vi "AlliGator Close White Light Image.vi"(7 "AlliGator Ctrl Refnums":T1, 8 "error in (no error)":errorcluster, 11 "AlliGator IV DVR in":refnum<data-value>) -> (0 "error out":errorcluster, 1 "Message":string, 3 "AlliGator IV DVR out":refnum<data-value>)   [LabVIEW 2021, in "AlliGator Files.lvlib"]
doc: "Clears White Light Image structure."
uses:
  AlliGator Files.lvlib
  Internal Variables/AlliGator Internal Variables v2.ctl
  <vilib>/vision/Image Controls.llb/IMAQ Image.ctl
  Internal Variables/AlliGator Gate Image Set.ctl
  AlliGator FLI Dataset Type.ctl
  AlliGator Data Series Type.ctl
  Dual-Channel Datasets/AlliGator Dataset Channel.ctl
  Settings/AlliGator Gate Arithmetic.ctl
  Source Image/AlliGator Displayed Image.ctl
  Image/Named ROI Description.ctl
  Phasor Graph/AlliGator Decay Metadata v3.ctl
  Decay Analysis/Decay Preprocessing/AlliGator Decay Background Subtraction Info.ctl
  Decay Analysis/Decay Preprocessing/AlliGator Baseline Subtraction Method.ctl
  Graphs/XY Graph/XY Graph Plot Shift Parameters.ctl
  Graphs/XY Graph/XY Graph Plot Shift Method.ctl
  Decay Analysis/Decay Preprocessing/AlliGator Decay Extrapolation Parameters.ctl
  Phasor/Calibration Phasor (m, phi).ctl
  Phasor/Phasor Reference Series.ctl
  Phasor/Phasor Calibration Map v2.ctl
  Phasor/Phasor (g, s).ctl
  Phasor Graph/AlliGator Raw Phasor Plot Data v5.ctl
  Phasor/Phasor Standard Deviation Options.ctl
  Phasor Plot/AlliGator Phasor Multi-Harmonic Data.ctl
  Phasor/Phasor Harmonic Data.ctl
  Decay Fit Parameter Map/AlliGator Decay Fit Options & Parameters v3.ctl
  Fits/IRF(X)PSED/Decay Fit Options v3.ctl
  Fits/Decay Convolution/Decay Model.ctl
  Fits/Residual Type.ctl
  Fits/IRF(X)PSED/Fit Weights Type.ctl
  Fits/Non-linear Fitting Method v2.ctl
  Fits/Fit Calculation Method.ctl
  Fits/Non-linear Fitting Algorithm.ctl
  Decay Analysis/Decay Fit/AlliGator Decay Fit Parameter Constraints 2.ctl
  Fits/IRF(X)PSED/Decay Fit Parameters In List.ctl
  Fits/IRF(X)PSED/MLE Baseline Offset Type.ctl
  Decay Analysis/Decay Preprocessing/AlliGator Decay Preprocessing Parameters.ctl
  Fits/IRF(X)PSED/Decay Fit Parameters & Derived Quantities List v2.ctl
  Fits/IRF(X)PSED/Decay Fit Result Constraint.ctl
  Decay Fit Parameter Map/AlliGator Parameter Maps Data.ctl
  GUI/AlliGator Ctrl Refnums.ctl
  GUI/AlliGator Other Ctrl Refnums.ctl
  GUI/AlliGator State Indicator.ctl
  GUI/AlliGator Main Window Tabs.ctl
  GUI/AlliGator Phasor Plot Ctrl Refnums.ctl
  GUI/AlliGator Phasor Graph Ctrl Refnums.ctl
  Phasor/Phasor Calibration Type.ctl
  GUI/AlliGator Dataset Ctrl Refnums.ctl
  GUI/AlliGator Registered Events Ctrl Refnums.ctl
  GUI/AlliGator Image Histogram Control Refnums.ctl
  Histograms/Linear Histogram Options.ctl
  Histograms/Histogram Bin Option.ctl
  Histograms/Histogram Bin Position.ctl
  Decay Fit Parameter Map/AlliGator Decay Fit Map Control Refnums.ctl
  Parameter Map/AlliGator Parameter Map Control Refnums.ctl
  Phasor/Phasor.lvlib
  Image/Image.lvlib
  Decay Analysis/Decay Preprocessing/AlliGator Decay Preprocessing.lvlib
  Phasor Graph/AlliGator Phasor Graph.lvlib
  Internal Variables/AlliGator Internal Variables.lvlib
  Phasor Plot/AlliGator Phasor Plot.lvlib
  Source Image/AlliGator Source Image.lvlib
  Fits/Fits.lvlib
  Decay Analysis/Decay Fit/AlliGator Decay Fit.lvlib
  Decay Fit Parameter Map/AlliGator Decay Fit Parameter Map.lvlib
  Settings/AlliGator Settings.lvlib
  Dual-Channel Datasets/AlliGator Dual-Channel Datasets.lvlib
  GUI/AlliGator GUI.lvlib
  Histograms/Histogram Window.lvlib
  Graphs/XY Graph/XY Graph Add-Ons.lvlib
  Parameter Map/AlliGator Parameter Map.lvlib
panel:
  # "see the AlliGator License on the block diagram (Ctrl+E or Window:Show Block Diagram)"
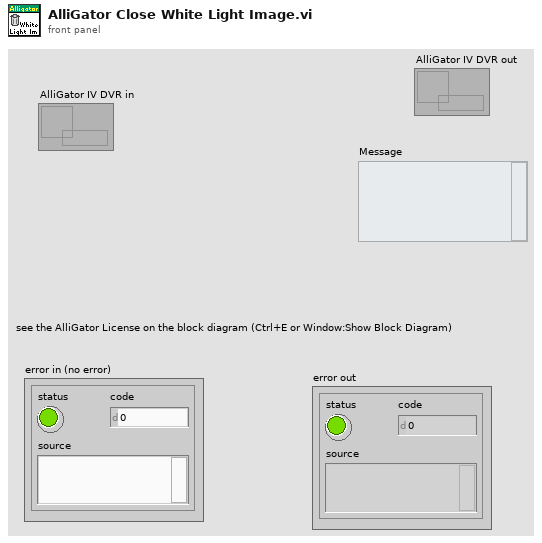
[diagram p1: front panel]
types:
  T1 = typedef "AlliGator GUI.lvlib/AlliGator Ctrl Refnums.ctl" = cluster{"Other AlliGator Ctrl Refnums":T2, "Phasor Plot Ctrl Refnums":T3, "Phasor Graph Ctrl Refnums":T4, "Dataset Control Refnums":T5, "Registered Events Ctrl Refnums":T6, "Image Histogram Ctrl Refnums":T7, "Decay Fit Map Ctrl Refnums":T8, "Parameter Map Ctrl Refnums":T9}
  T2 = typedef "AlliGator GUI.lvlib/AlliGator Other Ctrl Refnums.ctl" = cluster{"State Indicators":refnum<vi>, " Progress Bar":refnum<vi>, "Decay Graph Active":refnum<vi>, "Decay Statistics Bin":refnum<vi>, "Time Step":refnum<vi>, "Use File Timestamp":refnum<vi>, "Tab Control":refnum<vi>, "CPU":refnum<vi>, "Abort Fit":refnum<vi>, "Dataset File/Folder Path":refnum<vi>, "Abort ROI Creation":refnum<vi>, "Event LED":refnum<vi>, "Dataset File/Folder Path 2":refnum<vi>, "Dataset File/Folder Path 3":refnum<vi>, "Dataset File/Folder Path 4":refnum<vi>, "Dataset File/Folder Path 5":refnum<vi>, "Dataset File/Folder Path 6":refnum<vi>, "Dataset File/Folder Path 7":refnum<vi>, "Dataset File/Folder Path 8":refnum<vi>, "Dataset File/Folder Path 9":refnum<vi>, "Dataset File/Folder Path 10":refnum<vi>, "Dataset File/Folder Path 11":refnum<vi>}
  T3 = typedef "AlliGator GUI.lvlib/AlliGator Phasor Plot Ctrl Refnums.ctl" = cluster{"Phasor Ratio":refnum<vi>, "Modulus Lifetime":refnum<vi>, "Phasor at cursor (m, phi)":refnum<vi>, "Phase Lifetime":refnum<vi>, "Phasor at cursor (g, s)":refnum<vi>, "Phasor Plor Average Lifetime":refnum<vi>, "Phasor Plot Active":refnum<vi>, "Save Phasor Plot":refnum<vi>, "Image Overlay Color":refnum<vi>, "Phasor Plot Color Scale":refnum<vi>, "Reference 1 Button":refnum<vi>, "Reference 2 Button":refnum<vi>, "True Phasor Plot Value":refnum<vi>}
  T4 = typedef "AlliGator GUI.lvlib/AlliGator Phasor Graph Ctrl Refnums.ctl" = cluster{"Phasor Ratio":refnum<vi>, "Modulus Lifetime":refnum<vi>, "Phasor at cursor (m, phi)":refnum<vi>, "Phase Lifetime":refnum<vi>, "Phasor at cursor (g, s)":refnum<vi>, "Phasor Graph Average Lifetime":refnum<vi>, "Phasor Graph Active":refnum<vi>, "Save Phasor Graph":refnum<vi>, "Phasor Frame Slide":refnum<vi>, "Single Step Phasor":refnum<vi>, "Calibration Type":refnum<vi>, "Show Line":refnum<vi>, "Phase Lifetime 1":refnum<vi>, "Phase Lifetime 2":refnum<vi>, "Phasor Graph Frequency":refnum<vi>, "Phasor Reference 1 Control":refnum<vi>, "Phasor Reference 2 Control":refnum<vi>, "Calibration Lifetime":refnum<vi>, "Phase Lifetime SDV":refnum<vi>, "Average Lifetime SDV":refnum<vi>, "Phasor Ratio SDV":refnum<vi>, "Modulus Lifetime SDV":refnum<vi>}
  T5 = typedef "AlliGator GUI.lvlib/AlliGator Dataset Ctrl Refnums.ctl" = cluster{"Current Data":refnum<vi>, "Gate Image Slide":refnum<vi>, "Time Point Slide":refnum<vi>, "Current Time Stamp":refnum<vi>, "Save Image":refnum<vi>, "Displayed Image":refnum<vi>, "Overlay Mode":refnum<vi>, "Phasor Overlay Color":refnum<vi>, "Image Color Scale":refnum<vi>, "Use ROI as Search Area":refnum<vi>, "Source Image ROI Color":refnum<vi>, "True Pixel Value":refnum<vi>}
  T6 = typedef "AlliGator GUI.lvlib/AlliGator Registered Events Ctrl Refnums.ctl" = cluster{"Time Point Slider":refnum<vi>, "Phasor Plot Display Range":refnum<vi>, "Decay Graph":refnum<vi>, "Decay Statistics Graph":refnum<vi>, "Intensity Time Trace":refnum<vi>, "Phasor Graph":refnum<vi>, "Phasor Ratio Graph":refnum<vi>, "Lifetime Graph":refnum<vi>, "Phasor Plot Display":refnum<vi>, "Source Image Display":refnum<vi>, "Decay Fit Parameter Map Display Range":refnum<vi>, "Decay Fit Parameter Map Display":refnum<vi>, "Parameter Map Display Range":refnum<vi>, "Parameter Map Display":refnum<vi>, "Phasor Plot Display Range":refnum<vi>}
  T7 = typedef "AlliGator GUI.lvlib/AlliGator Image Histogram Control Refnums.ctl" = cluster{"Image Histogram":refnum<vi>, "Image Histogram Options":refnum<vi>, "Image Histogram Active":refnum<vi>, "Image Histogram Upper Percentile":refnum<vi>, "Image Histogram Lower Percentile":refnum<vi>, "Auto-Adjust Contrast":refnum<vi>}
  T8 = typedef "AlliGator Decay Fit Parameter Map.lvlib/AlliGator Decay Fit Map Control Refnums.ctl" = cluster{"Decay Fit Parameter Map Color Scale":refnum<vi>, "Decay Fit Parameter":refnum<vi>, "Max Parameter":refnum<vi>, "Min Parameter":refnum<vi>, "Decay Fit Parameter Map Display":refnum<vi>, "Decay Fit Parameter Map Display Range":refnum<vi>, "Decay Parameter Map X":refnum<vi>, "Decay Parameter Map Y":refnum<vi>, "Decay Parameter Map Value":refnum<vi>}
  T9 = typedef "AlliGator Parameter Map.lvlib/AlliGator Parameter Map Control Refnums.ctl" = cluster{"Parameter Map Color Scale":refnum<vi>, "Map Parameter":refnum<vi>, "Max Parameter":refnum<vi>, "Min Parameter":refnum<vi>, "Parameter Map Display":refnum<vi>, "Parameter Map Display Range":refnum<vi>, "Parameter Map Set":refnum<vi>, "Parameter Map X":refnum<vi>, "Parameter Map Y":refnum<vi>, "Parameter Map Value":refnum<vi>}
  T10 = typedef "IMAQ Image.ctl" = refnum<image>
  T11 = typedef "AlliGator Internal Variables.lvlib/AlliGator Internal Variables v2.ctl" = cluster{"----------------------------- Images -----------------------------":u8, "Displayed Image":T10, "White Light Image":T10, "Mask Image":T10, "ROI Mask Image":T10, "Current Dataset Images 1":T12, "Background Dataset Images 1":T12, "Current Dataset Images 2":T12, "Background Dataset Images 2":T12, "Current Dataset Arithmetic Images":T12, "Accumulated Dataset Images 1":T12, "Accumulated Dataset Images 2":T12, "Accumulated Dataset Arithmetic Images":T12, "----------------------------- File Paths -----------------------------":u8, "Phasor Plot Image":T10, "Decay Fit Parameter Map Image":T10, "Parameter Map Image":T10, "Single Data Point Path":path, "White Light Image Path":path, "Mask Image Path":path, "Time-Series Folder":path, "[Time-Series Paths]":path[], "----------------------------- FLI Dataset -----------------------------":u8, "Current Dataset":i32, "Single Dataset Type":T13, "Current Folder":string, "AlliGator Data Series Type":T14, "# Datasets":i32, "Dual-Channel Dataset":bool, "Selected Channel Name":string, "Dataset Channel":T15, "Channel Arithmetic":T16, "Dual-Channel Background Dataset":bool, "Background Channel":T15, "Dual-Channel Accumulated Dataset":bool, "Start Time":dbl, "[Time-Series Timestamps]":dbl[], "[Intensity Corrections]":dbl[], "Time Series Script":bool, "Type of Displayed Image":T17, "Gate Image Slide":u16, "# Gates":i32, "ROIs":T18[], "----------------------------- Decays -----------------------------":u8, "ROI Decay":cluster{"t Array":dbl[], "I Array":dbl[]}, "Valid Decay":bool, "Decay  Metadata":T20, "Reference Decay Plot Name":string, "Reference Decay":cluster{"t Array":dbl[], "I Array":dbl[]}, "Decay Shift Plot":cluster{"Time Stamps":dbl[], "Decay Shifts":dbl[]}, "[Decays Max Values]":sgl[], "[Decays Min Values]":sgl[], "----------------------------- Calibration -----------------------------":u8, "Calibration Phasor":T26, "Calibration Phasor Series":T27, "Phasor Calibration Map":T28, "Calibration Map MD5 Digest":string, "----------------------------- Phasor Graph -----------------------------":u8, "Last Raw Phasor":T29, "Last Calibrated Phasor":T29, "Last Calibrated Phasor SDV":T29, "Phasor Graph:Phasor Plot":cluster{"g Array":dbl[], "s Array":dbl[]}, "Phasor Graph:Phasor SDV Plot":cluster{"g Array":dbl[], "s Array":dbl[]}, "[Phasor Graph:Raw Phasor Plots]":T30[], "Phasor Plot locked to Ref 1":i32, "[Phasor Plot(s) locked to Ref 1]":i32[], "[Phasor Plot(s) locked to Ref 2]":i32[], "[Pixel Phasors]":T29[], "----------------------------- Phasor Plot -----------------------------":u8, "[[Sum Image]]":dbl[][], "[[CSG Phasors]]":csg[][], "[[Valid Pixel?]]":bool[][], "[[Phasor Ratios]]":dbl[][], "[[Average Lifetimes]]":dbl[][], "Amplitude Weighted Average Lifetime":bool, "I/m/phi Dataset":cluster{"I/m/phi Dataset?":bool, "Base Frequency":dbl[unit], "Harmonic Orders":u8[]}, "Multi Phasor Plot Data":T32, "----------------------------- Decay Fit Parameter Map -----------------------------":u8, "Decay Fit Options & Parameters":T34, "Fit Options: Decay Preprocessing Parameters":T45, "Fit Options: Reference Decay":cluster{"t Array":dbl[], "I Array":dbl[]}, "Is Full Image Parameters Map":bool, "Is Single-Pixels Parameters Map":bool, "NLSF Parameters Map X Resolution":i32, "NLSF Parameters Map Y Resolution":i32, "[Single Decay Fit Parameters]":dbl[], "Fit Model":T36, "[[Multiple Decays Fit Parameters]]":dbl[][], "[[Multiple Decays Fit Parameter SDVs]]":dbl[][], "[[IRFs]]":dbl[][], "IRF Array Time Axis":dbl[], "Decay Array Time Axis":dbl[], "[Decay Fit Parameter Names]":T46[], "[Decay Sum]":dbl[], "Array of Decay Fit Result Constraints":T47[], "Selected ROIs Array":bool[], "----------------------------- Parameter Maps -----------------------------":u8, "[Map Set Names]":string[], "[Parameter Maps]":T48[], "[[User-defined Quantities]]":dbl[][], "User-defined Quantity":string}
  T12 = typedef "AlliGator Internal Variables.lvlib/AlliGator Gate Image Set.ctl" = cluster{"SGL Image Max":T10, "SGL Image Sum":T10, "SGL Gate Images":T10[], "SGL Image Min":T10}
  T13 = typedef "AlliGator Files.lvlib/AlliGator FLI Dataset Type.ctl" = enum16{"HDF5 FLI Dataset", "Gate Image Folder", ".sdt FLI Dataset (Becker & Hickl)", ".ptu FLI Dataset (PicoQuant)", "SS1 FLI Dataset", "SS2 FLI Dataset", "I/m/phi Dataset", ".bin FLI Dataset (PicoQuant Binned)", ".bin FLI Dataset (Piccolo Binned)", ".mat FLI Dataset"}
  T14 = typedef "AlliGator Files.lvlib/AlliGator Data Series Type.ctl" = enum16{"Not a Supported Series", "Gate Images Folder Series", "SwissSPAD 2 Dataset Series", "B&H FLI Dataset Series", "PicoQuant PTU FLI Dataset Series", "PicoQuant BIN FLI Dataset Series", "Piccolo hist BIN FLI Dataset Series", "HDF5 FLI Dataset Series"}
  T15 = typedef "AlliGator Dual-Channel Datasets.lvlib/AlliGator Dataset Channel.ctl" = enum16{"G2", "INT"}
  T16 = typedef "AlliGator Settings.lvlib/AlliGator Gate Arithmetic.ctl" = enum16{"None", "INT-G2", "G2/INT*<INT>", "(1 - G2/INT)*<INT>"}
  T17 = typedef "AlliGator Source Image.lvlib/AlliGator Displayed Image.ctl" = enum16{"Single Gate", "Sum of All Gates", "Max of All Gates", "Min of All Gates", "-", "White Ligth Image", "Mask Image"}
  T18 = typedef "Image.lvlib/Named ROI Description.ctl" = cluster{"ROI Descriptor":T19, "ROI Name":string, "Overlay Color":u32}
  T19 = typedef "ROI Descriptor" = cluster{"Global Rectangle":i32[], "Contours":cluster{"ID":enum32{"External", "Internal"}, "Type":u32, "Coordinates":i32[]}[]}
  T20 = typedef "AlliGator Phasor Graph.lvlib/AlliGator Decay Metadata v3.ctl" = cluster{"ROI Descriptor":T19, "ROI Center":cluster{"X":i32, "Y":i32}, "Decay Background Subtraction Info":T21, "Decay Reverted":bool, "Decay Smoothened":bool, "Decay Straightened":bool, "Fitted Tau (Decay Straightening)":dbl, "Decay Shift Parameters":T23, "Decay Shifted":bool, "Decay Extrapolated":bool, "Decay Extrapolation Parameters":T25, "Decay Normalized":bool, "Fold Decay":bool, "# Folds":u32}
  T21 = typedef "AlliGator Decay Preprocessing.lvlib/AlliGator Decay Background Subtraction Info.ctl" = cluster{"Laser Period":dbl[unit], "Gate Duration":dbl[unit], "Baseline Subtraction Method":T22, "Background Definition Range":cluster{"Min Gate":dbl[unit], "Max Gate":dbl[unit]}, "Total Intensity w/o Bkgd Subtraction":dbl, "Bkgd-subtracted Intensity (exp)":dbl, "# Data Points":i32, "Background/Gate":dbl, "Fitted Lifetime":dbl[unit], "Bkgd-subtracted Intensity (theo)":dbl}
  T22 = typedef "AlliGator Decay Preprocessing.lvlib/AlliGator Baseline Subtraction Method.ctl" = enum16{"Mean", "Min", "Square Gated Single-Exponential", "File", "Constant"}
  T23 = typedef "XY Graph Add-Ons.lvlib/XY Graph Plot Shift Parameters.ctl" = cluster{"Type":T24, "Shift":dbl[unit], "Threshold":dbl, "Rotate":bool}
  T24 = typedef "XY Graph Add-Ons.lvlib/XY Graph Plot Shift Method.ctl" = enum16{"Default", "CFD", "Threshold", "Cross-Correlation"}
  T25 = typedef "AlliGator Decay Preprocessing.lvlib/AlliGator Decay Extrapolation Parameters.ctl" = cluster{"Additional Points":u32, "Head Fraction":dbl, "Fitted Tau":dbl, "Use Periodicity":bool, "Use Cursors":bool, "Tail Fraction":dbl}
  T26 = typedef "Phasor.lvlib/Calibration Phasor (m, phi).ctl" = cluster{"m":dbl, "phi":dbl, "Phasor Frequency":dbl[unit], "Reference Lifetime":dbl[unit]}
  T27 = typedef "Phasor.lvlib/Phasor Reference Series.ctl" = cluster{"m Array":dbl[], "phi Array":dbl[], "Phasor Frequency":dbl[unit], "Calibration Lifetime":dbl[unit]}
  T28 = typedef "Phasor.lvlib/Phasor Calibration Map v2.ctl" = cluster{"Phasor Frequency":dbl[unit], "Calibration Lifetime":dbl[unit], "ROI Centers":cluster{"X":i32, "Y":i32}[], "ROI Descriptors":T19[], "Map Resolution X":i32, "Map Resolution Y":i32, "z Array":cdb[]}
  T29 = typedef "Phasor.lvlib/Phasor (g, s).ctl" = cluster{"g":dbl, "s":dbl}
  T30 = typedef "AlliGator Phasor Graph.lvlib/AlliGator Raw Phasor Plot Data v5.ctl" = cluster{"Phasor Plot Name":string, "Raw Phasor Plot":T29[], "Phasor Frequency":dbl[unit], "[Decay Metadata]":T20[], "Raw Phasor Plot SDV":T29[], "Phasor SDV Options":T31, "[Calibration Phasor]":T26[], "Intensity Array":dbl[]}
  T31 = typedef "Phasor.lvlib/Phasor Standard Deviation Options.ctl" = cluster{"Compute Estimated SDV":bool, "# Replicas":u32, "Use Estimated Average Phasor":bool}
  T32 = typedef "AlliGator Phasor Plot.lvlib/AlliGator Phasor Multi-Harmonic Data.ctl" = cluster{"Base Frequency":dbl[unit], "# Harmonics":u8, "Harmonic Orders":u8[], "Phasor Plot Settings Checksum":u64, "Phasor Harmonic Data Array":T33[]}
  T33 = typedef "Phasor.lvlib/Phasor Harmonic Data.ctl" = cluster{"Phasor Harmonic Name":string, "Phasor Plot Settings Checksum":u64, "Phasor Frequency":dbl[unit], "Base Frequency":dbl[unit], "Harmonic Order":u8, "Phasor Plot Parameters":string, "Phasor Array [[CSG]]":csg[][], "Dataset File Path":path}
  T34 = typedef "AlliGator Decay Fit Parameter Map.lvlib/AlliGator Decay Fit Options & Parameters v3.ctl" = cluster{"SYNC Period":dbl[unit], "Fit Options":T35, "Fit Parameter Constraints":T42[], "MLE Baseline Offset":dbl, "MLE Baseline Offset Type":T44}
  T35 = typedef "Fits.lvlib/Decay Fit Options v3.ctl" = cluster{"Show Fit Residuals":bool, "Fit Model":T36, "Residual Type":T37, "Max Decay Percentile":dbl, "Min Decay Percentile":dbl, "Show Full Decay":bool, "Weights":T38, "Fitting Method":T39, "Compute Parameter Uncertainties":bool, "Periodic Boundaries":bool, "Model Calculation":T40, "Period":dbl[unit], "Termination Criteria":cluster{"Max Iterations":i32, "Max Function Calls":i32, "Max Time":dbl[unit], "Function Tolerance":dbl, "Parameter Tolerance":dbl, "Gradient Tolerance":dbl, "Min Lambda":dbl, "Max Lambda":dbl, "Initial Tick Count":u32}, "Offset Resolution":dbl[unit], "Use Local IRF":bool, "Fitting Algorithm":T41, "Show Confidence Interval ":bool, "Confidence Level":dbl}
  T36 = typedef "Fits.lvlib/Decay Model.ctl" = enum16{"1-Exponential", "2-Exponentials"}
  T37 = typedef "Fits.lvlib/Residual Type.ctl" = enum16{"Standard", "Normalized", "Reduced"}
  T38 = typedef "Fits.lvlib/Fit Weights Type.ctl" = enum16{"Unweighted", "1/Variance", "Best of All"}
  T39 = typedef "Fits.lvlib/Non-linear Fitting Method v2.ctl" = enum16{"Least Square", "Least Absolute Residual", "Bisquare", "MLE", "-", "Best of All"}
  T40 = typedef "Fits.lvlib/Fit Calculation Method.ctl" = enum16{"Simulation", "Convolution", "Integration"}
  T41 = typedef "Fits.lvlib/Non-linear Fitting Algorithm.ctl" = enum16{"Levenberg-Marquardt", "Trust-Region Dogleg"}
  T42 = typedef "AlliGator Decay Fit.lvlib/AlliGator Decay Fit Parameter Constraints 2.ctl" = cluster{"Fit Parameter":T43, "Min Value":dbl, "Max Value":dbl, "Global":bool, "Used":bool}
  T43 = typedef "Fits.lvlib/Decay Fit Parameters In List.ctl" = enum16{"Offset", "Baseline", "A_1", "tau_1", "A_2", "tau_2"}
  T44 = typedef "Fits.lvlib/MLE Baseline Offset Type.ctl" = enum32{"Absolute", "Percentage"}
  T45 = typedef "AlliGator Decay Preprocessing.lvlib/AlliGator Decay Preprocessing Parameters.ctl" = cluster{"Background Subtraction":bool, "Straighten Decay":bool, "Reverse Gates":bool, "1-Normalized Decay":bool, "Smoothen Decay":bool, "Smoothing Parameter":dbl, "Shift Decay":bool, "Decay Shift Parameters":T23, "Extrapolate Decay":bool, "Additional Points":u32, "Head Fraction":dbl, "Pixel-Normalize Decay":bool, "Use Periodicity":bool, "Use Cursors":bool, "Tail Fraction":dbl, "Use Decay Pre-Processing":bool, "Fold Decay":bool, "# Folds":u32, "[0-1]-Normalized Decay":bool}
  T46 = typedef "Fits.lvlib/Decay Fit Parameters & Derived Quantities List v2.ctl" = enum16{"Offset", "Baseline", "A_1", "tau_1", "A_2", "tau_2", "<tau>_a", "f1_a", "f2_a", "<tau>_i", "f1_i", "f2_i", "-", "R^2", "Chi^2"}
  T47 = typedef "Fits.lvlib/Decay Fit Result Constraint.ctl" = cluster{"Fit Parameter":enum16{"Offset", "Baseline", "A_1", "tau_1", "A_2", "tau_2", "<tau>_a", "f1_a", "f2_a", "<tau>_i", "f1_i", "f2_i", "-", "R^2", "Chi^2", "Max Relative Residual", "<Residual ACF>", "Residual ACF SDV", "tau_2/tau_1"}, "Min Value":dbl, "Max Value":dbl}
  T48 = typedef "AlliGator Decay Fit Parameter Map.lvlib/AlliGator Parameter Maps Data.ctl" = cluster{"Map Set Name":string, "[Parameter Names]":string[], "[[Parameters]]":dbl[][], "[[Parameter SDVs]]":dbl[][], "Decay Array Time Axis":dbl[], "[[IRFs]]":dbl[][], "IRF Array Time Axis":dbl[], "X Resolution":i32, "Y Resolution":i32, "Intensity Array":dbl[]}
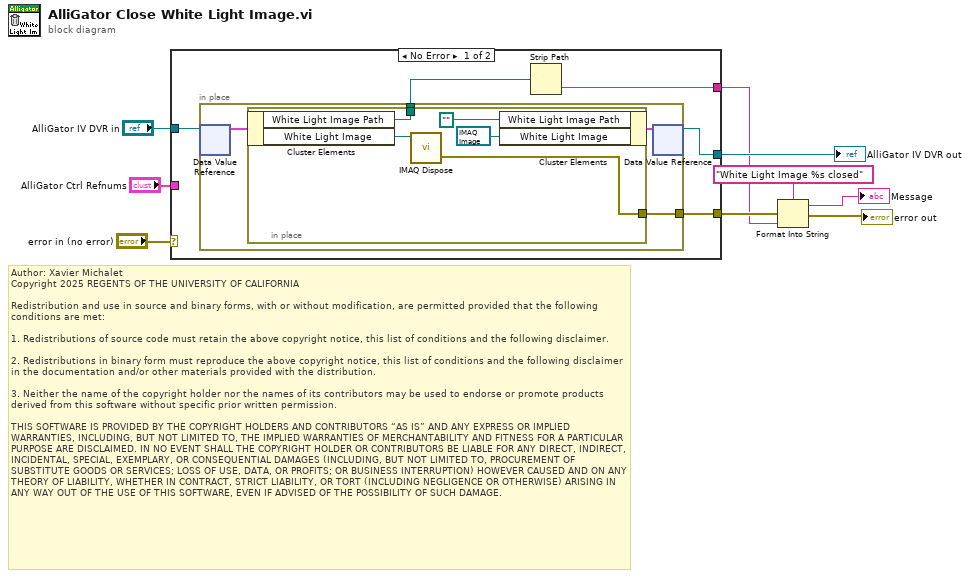
[diagram p0: block diagram]
diagram:
  # "Author: Xavier Michalet\nCopyright 2025 REGENTS OF THE UNIVERSITY OF CALIFORNIA\n\nRedistribution and use in source and binary forms, with or without modification, are permitted provided that the following conditions are met:\n\n1. Redistributions of source code must retain the above copyright notice, this list of conditions and the following disclaimer.\n\n2. Redistributions in binary form must reproduce the above copyright notice, this list of conditions and the following disclaimer in the documentation and/or other materials provided with the distribution.\n\n3. Neither the name of the copyright holder nor the names of its contributors may be used to endorse or promote products derived from this software without specific prior written permission.\n\nTHIS SOFTWARE IS PROVIDED BY THE COPYRIGHT HOLDERS AND CONTRIBUTORS “AS IS” AND ANY EXPRESS OR IMPLIED WARRANTIES, INCLUDING, BUT NOT LIMITED TO, THE IMPLIED WARRANTIES OF MERCHANTABILITY AND FITNESS FOR A PARTICULAR PURPOSE ARE DISCLAIMED. IN NO EVENT SHALL THE COPYRIGHT HOLDER OR CONTRIBUTORS BE LIABLE FOR ANY DIRECT, INDIRECT, INCIDENTAL, SPECIAL, EXEMPLARY, OR CONSEQUENTIAL DAMAGES (INCLUDING, BUT NOT LIMITED TO, PROCUREMENT OF SUBSTITUTE GOODS OR SERVICES; LOSS OF USE, DATA, OR PROFITS; OR BUSINESS INTERRUPTION) HOWEVER CAUSED AND ON ANY THEORY OF LIABILITY, WHETHER IN CONTRACT, STRICT LIABILITY, OR TORT (INCLUDING NEGLIGENCE OR OTHERWISE) ARISING IN ANY WAY OUT OF THE USE OF THIS SOFTWARE, EVEN IF ADVISED OF THE POSSIBILITY OF SUCH DAMAGE."
  n1 = case shown="No Error" "error in (no error)" {
    selector: "error in (no error)" -> [_ w25]
    tunnel: "AlliGator Ctrl Refnums" -> [_ _]
    tunnel: [w14 w24] -> w8
    tunnel: "AlliGator IV DVR in" -> [w13 w24]
    tunnel: [w12 w25] -> w5
    tunnel: [w10 _] -> w1
    frame No Error {
      n2 = in-place {
        in-place-border: [w16] -> w12
        in-place-border: [w15] -> w11
        n3 = in-place-dvr #1(w13) -> (w18:T11)  [unwired: 1 out]
        n4 = in-place {
          in-place-border: [w21] -> w16
          in-place-border: [w19] -> w15
          n5 = in-place-cluster #2(w18) -> ("White Light Image Path"=w19:path, "White Light Image"=w22:T10)
          n6 = call "IMAQ Dispose"("Image"=w22) -> ("error out"=w21:errorcluster)  [unwired: 5 in]
          n7 = in-place-cluster #2("White Light Image Path"=path "", "White Light Image"=T10 refnum) -> (w17:T11)
        }
        n8 = in-place-dvr #1(w17) -> (w14:refnum<data-value>)  [unwired: 1 out]
      }
      n9 = Strip Path(path=w11) -> (name=w10:string)  [unwired: 1 out]
    }
    frame Error {
    }
  }
  "AlliGator IV DVR out" <- w8
  n10 = Format Into String(format string="White Light Image %s closed", error in=w5, w1) -> (resulting string=→"Message":string, error out=→"error out":errorcluster)  [unwired: 1 in]
